vi "Comm_Receive(SubVI).vi"(7 "QueueSelector":T1, 8 "Error In":errorcluster) -> (0 "error out":errorcluster, 2 "Data":variant, 3 "Command":T2=enum."WaitOnReport")   [LabVIEW 2017, in "MainFrameLib.lvlib"]
uses:
  MainFrameLib.lvlib
  TypeDefs/Command_Enum.ctl
  TypeDefs/QNamesEnum.ctl
  TypeDefs/FGV_Enum.ctl
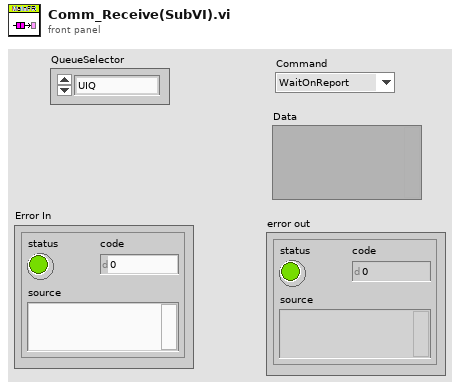
[diagram p1: front panel]
types:
  T1 = typedef "MainFrameLib.lvlib/QNamesEnum.ctl" = enum16{"UIQ", "ProcessQ", "CiscoQ", "KCSQ"}
  T2 = typedef "MainFrameLib.lvlib/Command_Enum.ctl" = enum16{"CheckSRLinks", "UpdateKCSColorCode", "StartLinkageCheck", "GetSRNotes", "DisplayAEStats", "InWork&Neglected", "RemapAENames", "ClearFolder", "UpdateReportsList", "ExcelReports", "TeamStats", "LoadReport", "WaitOnReport", "RequestReport", "Error", "Idle", "InitializeData", "ScreenPop", "Initialize", "UpdateCiscoAgentsView", "CancelRequests", "ClipboardCopy", "SaveNeglectedToFile", "Shutdown"}
  T3 = typedef "MainFrameLib.lvlib/FGV_Enum.ctl" = enum16{"Close", "GetRefs", "Initialize"}
  T4 = typedef "MainFrameLib.lvlib/DataCluster.ctl" = cluster{"Command":T2, "Data":variant}
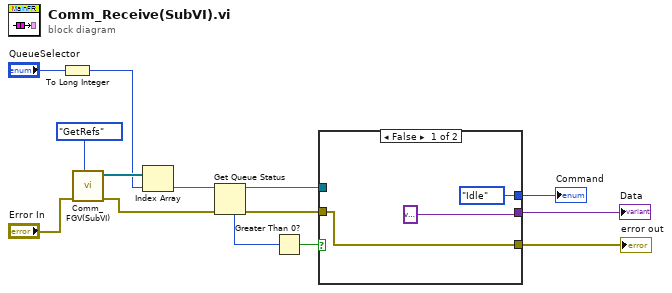
[diagram p0: block diagram]
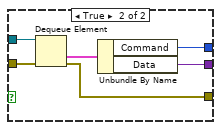
[diagram p2: hidden frame]
diagram:
  n1 = To Long Integer(number="QueueSelector") -> (32bit integer=w2:i32)
  n2 = call "Comm_FGV(SubVI).vi"("Enum"=FGV_Enum."GetRefs", "error in (no error)"="Error In") -> ("error out"=w10:errorcluster, "Array"=w5:refnum<queue>[])  [unwired: 8 in]
  n3 = Index Array(array=w5, index=w2) -> (element=w6:refnum<queue>)
  n4 = Get Queue Status(queue=w6, error in (no error)=w10) -> (queue out=w7:refnum<queue>, error out=w11:errorcluster, # elements in queue=w8:i32)  [unwired: 1 in, 5 out]
  n5 = Greater Than 0?(x=w8) -> (x > 0?=w9:bool)
  n6 = case shown="False" w9 {
    tunnel: w7 -> [_ w23]
    tunnel: w11 -> [w15 w22]
    tunnel: [Command_Enum."Idle" ("Command") w20] -> w12
    tunnel: [variant ("Data") w19] -> w13
    tunnel: [w15 w18] -> w14
    frame False {
    }
    frame True {
      n7 = Dequeue Element(queue=w23, error in (no error)=w22) -> (element=w21:T4, error out=w18:errorcluster)  [unwired: 1 in, 2 out]
      n8 = Unbundle By Name(w21) -> ("Command"=w20:T2, "Data"=w19:variant)
    }
  }
  "error out" <- w14
  "Data" <- w13
  "Command" <- w12
